vi "GetSurroundingPoints.vi"(10 "Accessors:Position (Tiles)":T1, 11 "AI_Snake in":refnum<class "AI_Snake.lvclass">) -> (2 "Array":T1[](array[typedef]), 3 "CycleValues":i16[](array[numeric]))   [LabVIEW 2019, in "RT_Game.lvlib" / "AI_Snake.lvclass"]
uses:
  AI_Snake.lvclass
  Engine/Coordinate.ctl
  Engine/Engine.lvclass
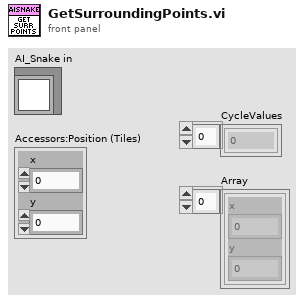
[diagram p1: front panel]
types:
  T1 = typedef "RT_Game.lvlib/Engine.lvclass/Coordinate.ctl" = cluster{"x":dbl, "y":dbl}
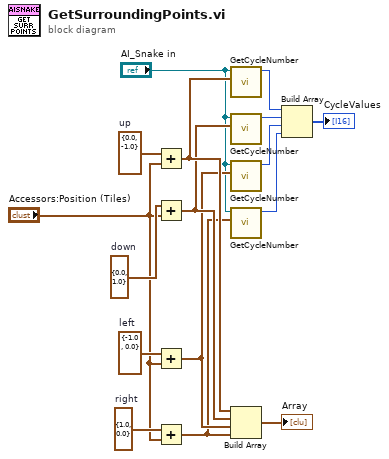
[diagram p0: block diagram]
diagram:
  w12 = T1 {"x"=0.0, "y"=-1.0}  # up
  w11 = T1 {"x"=0.0, "y"=1.0}  # down
  w10 = T1 {"x"=-1.0, "y"=0.0}  # left
  w9 = T1 {"x"=1.0, "y"=0.0}  # right
  n1 = Add(x=w12, y="Accessors:Position (Tiles)") -> (x+y=w15:T1)
  n2 = Add(x=w11, y="Accessors:Position (Tiles)") -> (x+y=w7:T1)
  n3 = Add(x=w10, y="Accessors:Position (Tiles)") -> (x+y=w5:T1)
  n4 = Add(x=w9, y="Accessors:Position (Tiles)") -> (x+y=w3:T1)
  n5 = call "GetCycleNumber.vi"("coordinate"=w15, "AI_Snake in"="AI_Snake in") -> ("CycleNumber"=w13:i16)  [unwired: 9 in]
  n6 = call "GetCycleNumber.vi"("coordinate"=w7, "AI_Snake in"="AI_Snake in") -> ("CycleNumber"=w6:i16)  [unwired: 9 in]
  n7 = call "GetCycleNumber.vi"("coordinate"=w5, "AI_Snake in"="AI_Snake in") -> ("CycleNumber"=w4:i16)  [unwired: 9 in]
  n8 = call "GetCycleNumber.vi"("coordinate"=w3, "AI_Snake in"="AI_Snake in") -> ("CycleNumber"=w1:i16)  [unwired: 9 in]
  n9 = Build Array(w15, w7, w5, w3) -> (→"Array":T1[])
  n10 = Build Array(w13, w6, w4, w1) -> (→"CycleValues":i16[])
